vi "TimeLeft.vi"(2 "I":u32, 3 "N":u32, 4 "Start Time":u32, 5 "End Time":u32) -> (0 "Time left ms":u32, 1 "Time Left String":string="0 hr 0 min 0 sec")   [LabVIEW 2012]
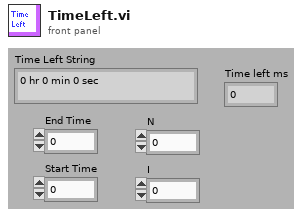
[diagram p1: front panel]
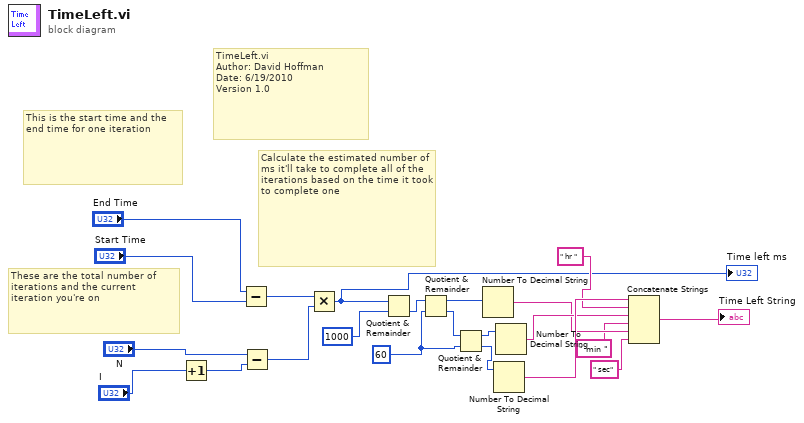
[diagram p0: block diagram]
diagram:
  w18 = 60
  # "TimeLeft.vi\nAuthor: David Hoffman\nDate: 6/19/2010\nVersion 1.0"
  # "Calculate the estimated number of ms it'll take to complete all of the iterations based on the time it took to complete one"
  # "This is the start time and the end time for one iteration"
  # "These are the total number of iterations and the current iteration you're on"
  n1 = Increment(x="I") -> (x+1=w8:u32)
  n2 = Subtract(x="End Time", y="Start Time") -> (x-y=w7:u32)
  n3 = Subtract(x="N", y=w8) -> (x-y=w6:u32)
  n4 = Multiply(x=w7, y=w6) -> (x*y=w1:u32)
  "Time left ms" <- w1
  n5 = Quotient & Remainder(x=w1, y=1000) -> (floor(x/y)=w21:u32)  [unwired: 1 out]
  n6 = Quotient & Remainder(x=w21, y=w18) -> (x-y*floor(x/y)=w20:u32, floor(x/y)=w19:u32)
  n7 = Quotient & Remainder(x=w19, y=w18) -> (x-y*floor(x/y)=w17:u32, floor(x/y)=w16:u32)
  n8 = Number To Decimal String(number=w20) -> (decimal integer string=w13:string)  [unwired: 1 in]
  n9 = Number To Decimal String(number=w16) -> (decimal integer string=w15:string)  [unwired: 1 in]
  n10 = Number To Decimal String(number=w17) -> (decimal integer string=w14:string)  [unwired: 1 in]
  n11 = Concatenate Strings(w15, " hr ", w14, " min ", w13, " sec") -> (→"Time Left String":string)
